vi "Cal Mic Sensitivity (TDT).vi"(8 "Device Config":T1, 9 "User ID":string, 10 "Mic Sens (dB V/SPL) in":dbl=-inf, 11 "Standalone":bool) -> (2 "Mic Sens (dB V/SPL)":dbl=-inf format="%.2f")   [LabVIEW 2020]
uses:
  epl-vi-lib/PXI DAQ VIs/TDT VIs/Typedefs/TDT-Device Config.ctl
  epl-vi-lib/PXI DAQ VIs/TDT VIs/Typedefs/TDT-Output source.ctl
  epl-vi-lib/PXI DAQ VIs/TDT VIs/Typedefs/TDT-Device ID.ctl
  epl-vi-lib/PXI DAQ VIs/TDT VIs/Typedefs/TDT-Input source.ctl
  Type Defs/ACal-Mic Sens Parameters.ctl
  epl-vi-lib/Utility VIs/Math VIs/Linear to dB (array).vi
  epl-vi-lib/Utility VIs/Conversion VIs/Create Waveform Cluster (1D).vi
  epl-vi-lib/Utility VIs/Math VIs/dB to Linear (scalar).vi
panel:
  out "mV/Pa":dbl=-inf format="%.2f"
  in  "Start":bool
  in  "Stop":bool
  in  "Return":bool
  out "Acquired":i32=4
  in  "Averages":i32=1
  in  "Sampling Rate (Hz)":dbl=20000.0
  in  "Pistonphone Output\n(dB SPL)":dbl=124.0 format="%.2f"
  in  "B&K Gain":dbl=40.0
  in  "Cal Log":path=path "C:/Data/Probe Tube Calibrations/Cal Mic Sensitivity Log.txt"
  out "calibrated":bool
  out "Log":string[][](table) caption="Calibration Log"
  out "abort":bool
  out "finished":errorcluster
  out "Magnitude":cluster{dbl, "dx":dbl, "Y":dbl[]}(graph)
  out "Waveform":dbl[](graph)
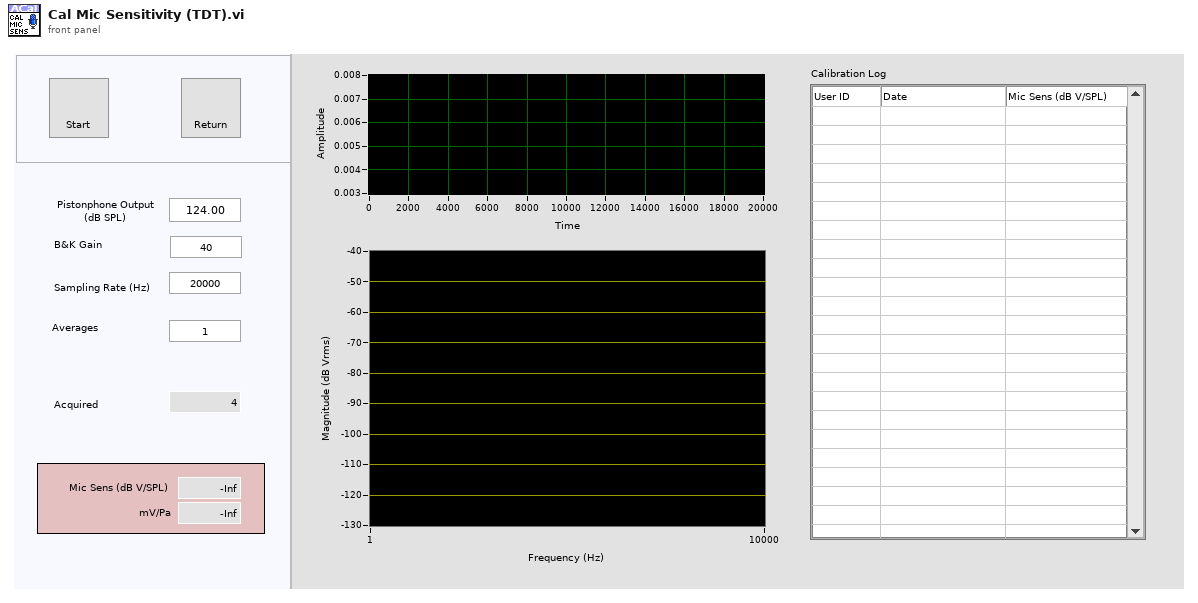
[diagram p1: front panel]
types:
  T1 = typedef "TDT-Device Config.ctl" = cluster{"Output":T2, "Input":T4}
  T2 = typedef "TDT-Output source.ctl" = cluster{"Device":T3, "Num":i32}
  T3 = typedef "TDT-Device ID.ctl" = enum16{"None", "PA5", "RP2", "RL2", "RA16", "RV8", "RX5", "RX6", "RX7", "RX8", "RZ2", "RZ5", "RZ6"}
  T4 = typedef "TDT-Input source.ctl" = enum16{"Front Panel", "RA4LI", "RA16LI"}
  T5 = typedef "ACal-Mic Sens Parameters.ctl" = cluster{"Pistonphone level (dB SPL)":dbl, "Sampling rate (Hz)":dbl, "Averages":i32, "Gain":dbl}
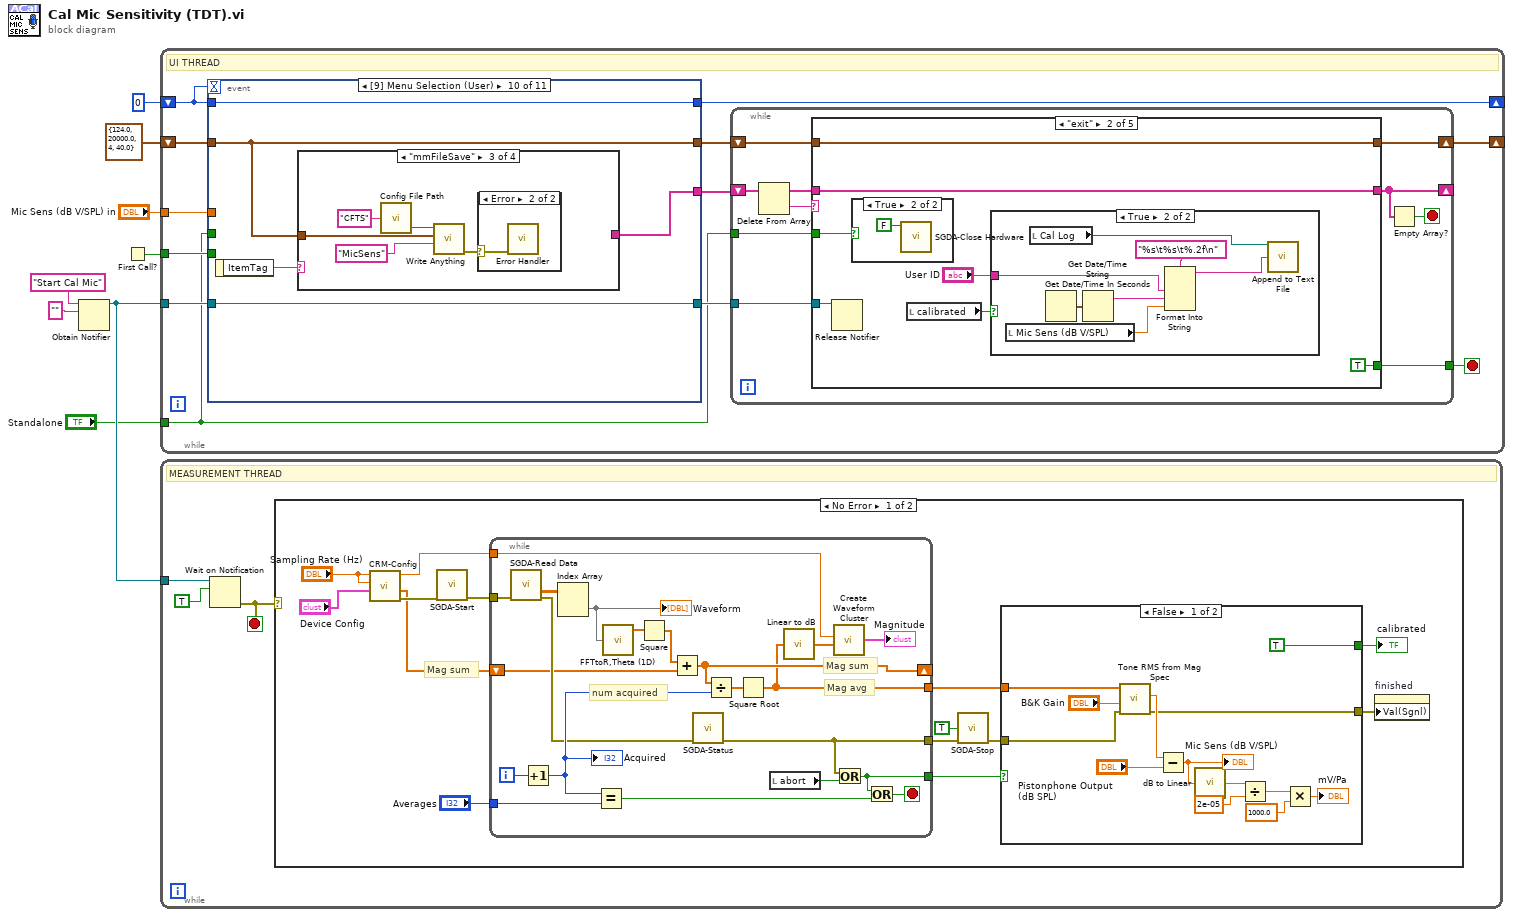
[diagram p0: block diagram]
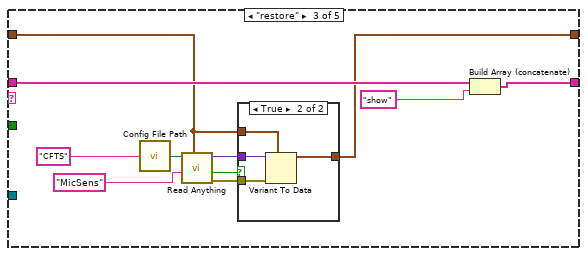
[diagram p7: hidden frame]
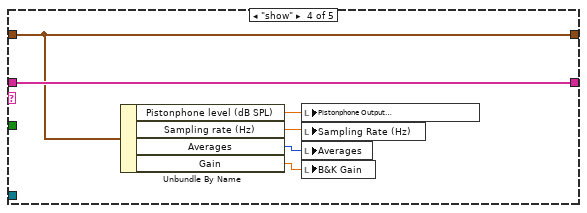
[diagram p9: hidden frame]
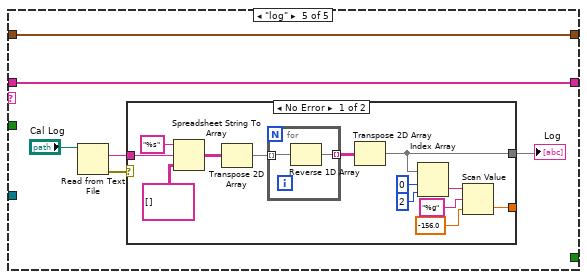
[diagram p10: hidden frame]
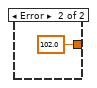
[diagram p11: hidden frame]
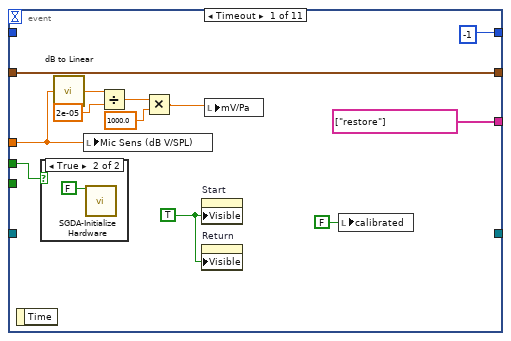
[diagram p12: hidden frame]
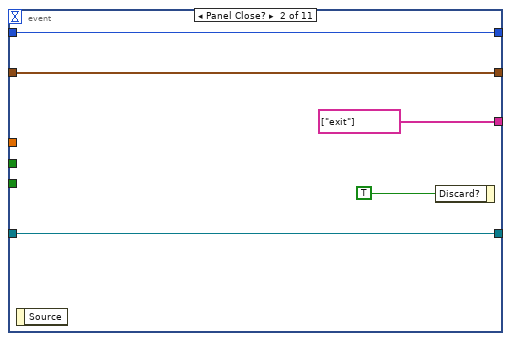
[diagram p14: hidden frame]
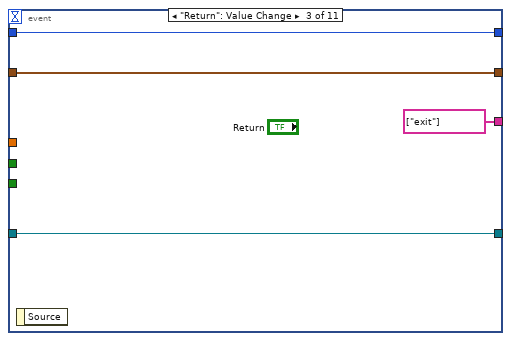
[diagram p15: hidden frame]
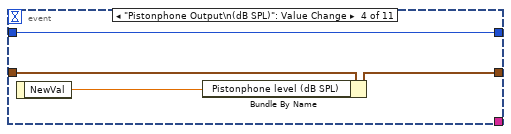
[diagram p16: hidden frame]
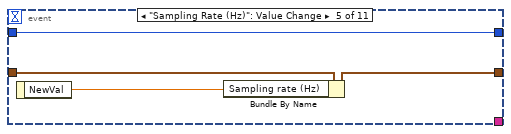
[diagram p17: hidden frame]
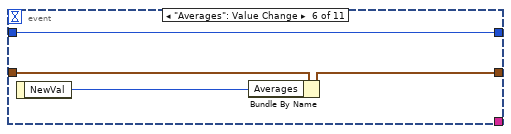
[diagram p18: hidden frame]
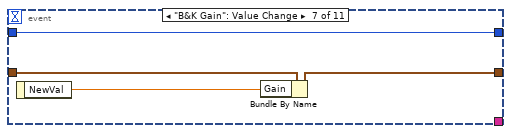
[diagram p19: hidden frame]
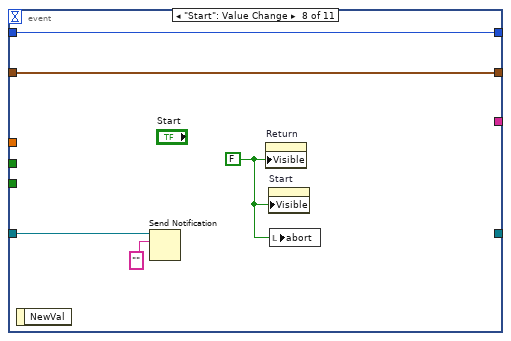
[diagram p20: hidden frame]
diagram:
  n1 = Obtain Notifier(name (unnamed)="Start Cal Mic", notification data type="") -> (notifier out=w8:refnum<notifier>)  [unwired: 2 in, 2 out]
  n2 = First Call?() -> (First Call?: T/F=w4:bool)
  n3 = while {
    tunnel: w8 -> [w20]
    shift-right: [w19] -> _
    shift-left: 0 -> [w16]
    tunnel: w4 -> [w18]
    tunnel: "Mic Sens (dB V/SPL) in" -> [w17]
    shift-right: [w11] -> _
    shift-left: T5 {"Pistonphone level (dB SPL)"=124.0, "Sampling rate (Hz)"=20000.0, "Averages"=4, "Gain"=40.0} ("Params") -> [w12]
    tunnel: "Standalone" -> [w9]
    stop <- w13 stop-if-true
    # "UI THREAD"
    n4 = event shown="[9] Menu Selection (User)" {
      selector: _ -> [_ _ _ _ _ _ _ _ _ _ _]
      dyn-events: _ -> [_ _ _ _ _ _ _ _ _ _ _]
      timeout: w16 -> [_ _ _ _ _ _ _ _ _ _ _]
      tunnel: w20 -> [_ w106 w113 _ _ _ _ w133 _ w140 _]
      tunnel: [_ w106 w113 _ _ _ _ _ _ w140 _] -> w14
      tunnel: [-1 w109 w112 w117 w121 w125 w129 w131 w137 w139 w155] -> w19
      tunnel: w18 -> [_ _ _ _ _ _ _ _ _ _ _]
      tunnel: w16 -> [_ w109 w112 w117 w121 w125 w129 w131 w137 w139 w155]
      tunnel: w17 -> [w93 _ _ _ _ _ _ _ _ _ _]
      tunnel: [string[] ["restore"] string[] ["exit"] string[] ["exit"] _ _ _ _ _ _ w141 _] -> w15
      tunnel: [w100 w105 w111 w115 w119 w123 w127 w130 w135 w138 w152] -> w10
      tunnel: w12 -> [w100 w105 w111 w116 w120 w124 w128 w130 w135 w138 w152]
      tunnel: w9 -> [w92 _ _ _ _ _ _ _ _ _ _]
      event Timeout {
        w102 = TRUE ("Visible")
        n5 = event-data() -> ()  [unwired: 1 in, 1 out]
        n6 = case shown="True" w92 {
          frame False {
          }
          frame True {
            n7 = call "SGDA-Initialize Hardware.vi"("Start PXI Server"=FALSE) -> ()  [unwired: 13 in, 2 out]
          }
        }
        n8 = call-poly "dB to Linear.vi"("dB"=w93) -> ("linear"=w98:dbl)
        n9 = local write "Mic Sens (dB V/SPL)"(w93) -> ()
        n10 = Divide(x=w98, y=2e-05) -> (x/y=w96:dbl)
        n11 = Multiply(x=w96, y=1000.0) -> (x*y=w94:dbl)
        n12 = property on="Start" class="Bool"("Visible"=w102) -> ()  [unwired: 2 in, 2 out]
        n13 = property on="Return" class="Bool"("Visible"=w102) -> ()  [unwired: 2 in, 2 out]
        n14 = local write "mV/Pa"(w94) -> ()
        n15 = local write "calibrated"(FALSE ("calibrated")) -> ()
      }
      event Panel Close? {
        n16 = event-data() -> ()  [unwired: 1 in, 1 out]
        n17 = event-data("Discard?"=TRUE) -> ()  [unwired: 1 in, 1 out]
      }
      event "Return": Value Change {
        n18 = event-data() -> ()  [unwired: 1 in, 1 out]
      }
      event "Pistonphone Output\n(dB SPL)": Value Change {
        n19 = event-data() -> ("NewVal"=w114:dbl)  [unwired: 1 in]
        n20 = Bundle By Name(cluster=w116, "Pistonphone level (dB SPL)"=w114) -> (w115:T5)
      }
      event "Sampling Rate (Hz)": Value Change {
        n21 = event-data() -> ("NewVal"=w118:dbl)  [unwired: 1 in]
        n22 = Bundle By Name(cluster=w120, "Sampling rate (Hz)"=w118) -> (w119:T5)
      }
      event "Averages": Value Change {
        n23 = event-data() -> ("NewVal"=w122:i32)  [unwired: 1 in]
        n24 = Bundle By Name(cluster=w124, "Averages"=w122) -> (w123:T5)
      }
      event "B&K Gain": Value Change {
        n25 = event-data() -> ("NewVal"=w126:dbl)  [unwired: 1 in]
        n26 = Bundle By Name(cluster=w128, "Gain"=w126) -> (w127:T5)
      }
      event "Start": Value Change {
        w132 = FALSE ("Visible")
        n27 = event-data() -> ()  [unwired: 1 in, 1 out]
        n28 = Send Notification(notification="", notifier=w133) -> ()  [unwired: 1 in, 2 out]
        n29 = property on="Return" class="Bool"("Visible"=w132) -> ()  [unwired: 2 in, 2 out]
        n30 = property on="Start" class="Bool"("Visible"=w132) -> ()  [unwired: 2 in, 2 out]
        n31 = local write "abort"(w132) -> ()
      }
      event "Stop": Value Change {
        n32 = event-data() -> ()  [unwired: 1 in, 1 out]
        "abort" <- TRUE ("abort")
      }
      event Menu Selection (User) {
        n33 = event-data() -> ("ItemTag"=w142:string)  [unwired: 1 in]
        n34 = case shown="\"mmFileSave\"" w142 {
          tunnel: [_ string[] ["restore"] _ string[] ["exit"]] -> w141
          tunnel: w138 -> [_ _ w144 _]
          frame "False", Default {
          }
          frame "mmFileRestore" {
          }
          frame "mmFileSave" {
            n35 = call "Config File Path.vi"("AppName"="CFTS") -> ("Default config file name"=w146:path)
            n36 = call "Write Anything.vi"("Section Name (Name of \"Anything\")"="MicSens" ("Section Name (Name of \"Type of Anything\")"), "Anything"=w144, "Path (dialog)"=w146) -> ("Error Out"=w145:errorcluster)  [unwired: 7 in, 1 out]
            n37 = case shown="Error" w145 {
              selector: w145 -> [_ w150]
              frame No Error {
                n38 = One Button Dialog(message="Defaults saved.") -> ()  [unwired: 1 in, 1 out]
              }
              frame Error {
                n39 = call "Error Handler.vi"("error in (no error)"=w150) -> ()  [unwired: 13 in, 2 out]
              }
            }
          }
          frame "mmFileExit" {
          }
        }
      }
      event "finished": Value Change {
        w154 = TRUE ("Visible")
        n40 = event-data() -> ("NewVal"=w153:errorcluster)  [unwired: 1 in]
        n41 = call "Error Handler.vi"("error in (no error)"=w153) -> ()  [unwired: 13 in, 2 out]
        n42 = property on="Start" class="Bool"("Visible"=w154) -> ()  [unwired: 2 in, 2 out]
        n43 = property on="Return" class="Bool"("Visible"=w154) -> ()  [unwired: 2 in, 2 out]
      }
    }
    n44 = while {
      shift-right: [w27] -> _
      shift-left: w15 -> [w30]
      tunnel: w14 -> [w25]
      tunnel: [w24] -> w13
      shift-right: [w23] -> w11
      shift-left: w10 -> [w22]
      tunnel: w9 -> [w21]
      stop <- w26 stop-if-true
      n45 = Delete From Array(array=w30) -> (deleted portion=w28:string, array with subset deleted=w29:string[])  [unwired: 2 in]
      n46 = case shown="\"exit\"" w28 {
        tunnel: w29 -> [w32 w39 w58 w69 w75]
        tunnel: [w32 w39 w57 w69 w75] -> w27
        tunnel: w25 -> [_ w38 _ _ _]
        tunnel: [_ TRUE _ _ _] -> w24
        tunnel: [w31 w36 w48 w68 w74] -> w23
        tunnel: w22 -> [w31 w36 w49 w68 w74]
        tunnel: w21 -> [_ w33 _ _ _]
        frame "", Default {
        }
        frame "exit" {
          n47 = Release Notifier(notifier=w38) -> ()  [unwired: 2 in, 3 out]
          n48 = case shown="True" w33 {
            frame False {
            }
            frame True {
              n49 = call "SGDA-Close Hardware.vi"("Stop PXI Server (T)"=FALSE) -> ()  [unwired: 6 in, 1 out]
            }
          }
          n50 = local read "calibrated"() -> (w34:bool)
          n51 = case shown="True" w34 {
            tunnel: "User ID" -> [_ w41]
            frame False {
            }
            frame True {
              n52 = local read "Mic Sens (dB V/SPL)"() -> (w46:dbl)
              n53 = local read "Cal Log"() -> (w43:path)
              n54 = Get Date/Time In Seconds() -> (seconds since 1Jan1904=w45:timestamp)
              n55 = Get Date/Time String(seconds (now)=w45) -> (date string=w47:string)  [unwired: 2 in, 1 out]
              n56 = Format Into String(format string="%s\t%s\t%.2f\n", w41, w47, w46) -> (resulting string=w44:string)  [unwired: 2 in, 1 out]
              n57 = call "Append to Text File.vi"("file path"=w43, "text"=w44) -> ()  [unwired: 12 in, 2 out]
            }
          }
        }
        frame "restore" {
          n58 = call "Config File Path.vi"("AppName"="CFTS") -> ("Default config file name"=w55:path)
          n59 = call "Read Anything.vi"("Type of Anything"=w49, "Section Name (Name of \"Type of Anything\")"="MicSens" ("Section Name (Name of \"Type of Anything\")"), "Path (dialog)"=w55) -> ("Error Out"=w51:errorcluster, "Found?"=w50:bool, "Anything"=w52:variant)  [unwired: 6 in]
          n60 = case shown="True" w50 {
            tunnel: w51 -> [_ w62]
            tunnel: w52 -> [_ w63]
            tunnel: w49 -> [w59 w61]
            tunnel: [w59 w60] -> w48
            frame False {
            }
            frame True {
              n61 = Variant To Data(error in=w62, type=w61, Variant=w63) -> (data=w60:T5)  [unwired: 1 out]
            }
          }
          n62 = Build Array (concatenate)(w58, "show") -> (w57:string[])
        }
        frame "show" {
          n63 = Unbundle By Name(w68) -> ("Pistonphone level (dB SPL)"=w67:dbl, "Sampling rate (Hz)"=w66:dbl, "Averages"=w65:i32, "Gain"=w64:dbl)
          n64 = local write "Pistonphone Output\n(dB SPL)"(w67) -> ()
          n65 = local write "Sampling Rate (Hz)"(w66) -> ()
          n66 = local write "Averages"(w65) -> ()
          n67 = local write "B&K Gain"(w64) -> ()
        }
        frame "log" {
          n68 = Read from Text File(file (use dialog)="Cal Log") -> (text=w70:string, error out=w71:errorcluster)  [unwired: 3 in, 2 out]
          n69 = case shown="No Error" w71 {
            tunnel: w70 -> [w88 _]
            tunnel: [w82 _] -> w73
            tunnel: [w78 102.0] -> _
            frame No Error {
              n70 = Spreadsheet String To Array(format string="%s", spreadsheet string=w88, array type (2D Dbl)=string[][] []) -> (array=w85:string[][])  [unwired: 1 in]
              n71 = Transpose 2D Array(2D array=w85) -> (transposed array=w84:string[][])
              n72 = for {
                tunnel: w84 -> [w90] mode=indexing
                tunnel: [w89] -> w83 mode=indexing
                n73 = Reverse 1D Array(array=w90) -> (reversed array=w89:string[])
              }
              n74 = Transpose 2D Array(2D array=w83) -> (transposed array=w82:string[][])
              n75 = Index Array(array=w82, index (row)=0, index (col)=2 ("disabled index (col)")) -> (element=w79:string)
              n76 = Scan Value(string=w79, format string="%g", default (0 dbl)=-156.0) -> (value=w78:dbl)  [unwired: 1 out]
            }
            frame Error {
            }
          }
          "Log" <- w73
        }
      }
      n77 = Empty Array?(array=w27) -> (empty?=w26:bool)
    }
  }
  n78 = while {
    tunnel: w8 -> [w157]
    stop <- w156 stop-if-true
    # "MEASUREMENT THREAD"
    n79 = Wait on Notification(notifier=w157, ignore previous (F)=TRUE) -> (error out=w156:errorcluster)  [unwired: 2 in, 3 out]
    n80 = case shown="No Error" w156 {
      frame No Error {
        # "Mag sum"
        n81 = call "CRM-Config.vi"("Device Config"="Device Config", "Num AI pts"="Sampling Rate (Hz)", "Sampling Rate (Hz)"="Sampling Rate (Hz)") -> ("error out"=w169:errorcluster, "Magnitude array"=w164:dbl[], "Freq resol (Hz)"=w165:dbl)  [unwired: 6 in]
        n82 = call "SGDA-Start.vi"("error in (no error)"=w169) -> ("error out"=w167:errorcluster)  [unwired: 6 in]
        n83 = while {
          tunnel: w167 -> [w207]
          tunnel: "Averages" -> [w205]
          tunnel: [w193] -> w170
          tunnel: [w187] -> w172
          shift-right: [w197] -> _
          shift-left: w164 -> [w196]
          tunnel: w165 -> [w199]
          tunnel: [w189] -> w162
          i -> [w206]
          stop <- w190 stop-if-true
          # "num acquired"
          # "Mag avg"
          # "Mag sum"
          n84 = call "SGDA-Read Data.vi"("error in (no error)"=w207) -> ("AI Waveforms"=w198:dbl[][], "error out"=w203:errorcluster)  [unwired: 13 in]
          n85 = Increment(x=w206) -> (x+1=w204:i32)
          "Acquired" <- w204
          n86 = Index Array(array=w198) -> (element=w194:dbl[])  [unwired: 2 in]
          "Waveform" <- w194
          n87 = Equal?(x=w204, y=w205) -> (x = y?=w191:bool)
          n88 = call "FFTtoR,Theta (1D).VI"("X"=w194) -> ("+Freq. Mag of FFT"=w195:dbl[])  [unwired: 1 in, 1 out]
          n89 = Square(x=w195) -> (x^2=w188:dbl[])
          n90 = Add(x=w188, y=w196) -> (x+y=w197:dbl[])
          n91 = call "SGDA-Status.vi"("error in (no error)"=w203) -> ("error out"=w193:errorcluster)  [unwired: 14 in]
          n92 = Divide(x=w197, y=w204) -> (x/y=w202:dbl[])
          n93 = Square Root(x=w202) -> (sqrt(x)=w187:dbl[])
          n94 = local read "abort"() -> (w192:bool)
          n95 = call-poly "Linear to dB.vi"("linear"=w187) -> ("dB"=w201:dbl[])
          n96 = call-poly "Create Waveform Cluster.vi"("dx"=w199, "Y"=w201) -> ("waveform cluster"=→"Magnitude":cluster{dbl, "dx":dbl, "Y":dbl[]})  [unwired: 3 in]
          n97 = Or(x=w193, y=w192) -> (x .or. y?=w189:bool)
          n98 = Or(x=w189, y=w191) -> (x .or. y?=w190:bool)
        }
        n99 = call "SGDA-Stop.vi"("Clear ActiveX (F)"=TRUE, "error in (no error)"=w170) -> ("error out"=w171:errorcluster)  [unwired: 13 in]
        n100 = case shown="False" w162 {
          tunnel: w172 -> [w185 _]
          tunnel: w171 -> [w184 w186]
          tunnel: [w181 w186] -> w163
          tunnel: [TRUE _] -> w160
          frame False {
            n101 = call "Tone RMS from Mag Spec.vi"("error in (no error)"=w184, "Gain"="B&K Gain", "Magnitude (dB)"=w185) -> ("error out"=w181:errorcluster, "RMS (dB)"=w183:dbl)  [unwired: 5 in, 2 out]
            n102 = Subtract(x=w183, y="Pistonphone Output\n(dB SPL)") -> (x-y=w174:dbl)
            "Mic Sens (dB V/SPL)" <- w174
            n103 = call-poly "dB to Linear.vi"("dB"=w174) -> ("linear"=w178:dbl)
            n104 = Divide(x=w178, y=2e-05) -> (x/y=w176:dbl)
            n105 = Multiply(x=w176, y=1000.0) -> (x*y=→"mV/Pa":dbl)
          }
          frame True {
          }
        }
        "calibrated" <- w160
        n106 = property on="finished" class="Clust (strict)"("Val(Sgnl)"=w163) -> ()  [unwired: 2 in, 2 out]
      }
      frame Error {
      }
    }
  }
